vi "LiveData.vi"() -> ()   [LabVIEW 2009]
panel:
  out "error out":errorcluster
  out "Waveform Graph":u16[](graph)
  in  "VISA resource name":refnum<visa-resource-name>="COM21"
  in  "stop":bool
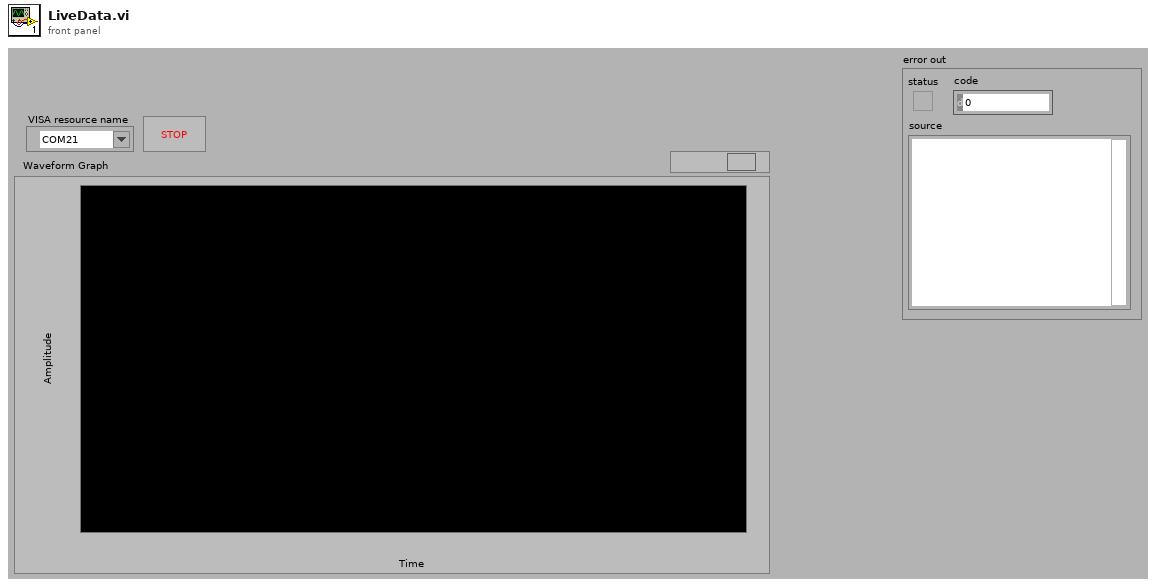
[diagram p1: front panel]
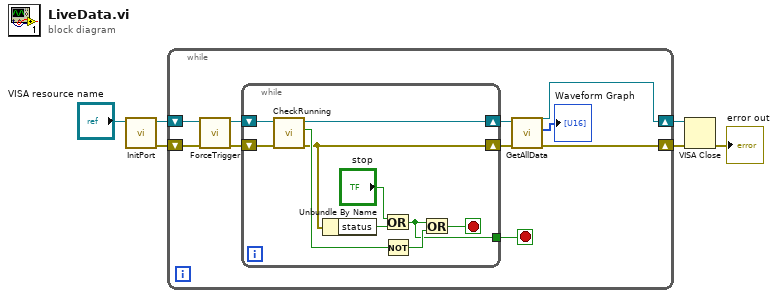
[diagram p0: block diagram]
diagram:
  n1 = call "InitPort.vi"("VISA resource name"="VISA resource name") -> ("error out"=w5:errorcluster, "VISA resource name out"=w4:refnum<visa-resource-name>)  [unwired: 9 in]
  n2 = while {
    shift-right: [w14] -> w3
    shift-left: w4 -> [w16]
    shift-right: [w13] -> w2
    shift-left: w5 -> [w15]
    stop <- w8 stop-if-true
    n3 = call "ForceTrigger.vi"("error in (no error)"=w15, "VISA resource name"=w16) -> ("error out"=w11:errorcluster, "VISA resource name out"=w12:refnum<visa-resource-name>)  [unwired: 8 in]
    n4 = while {
      shift-right: [w26] -> w10
      shift-left: w12 -> [w25]
      shift-right: [w21] -> w9
      shift-left: w11 -> [w24]
      tunnel: [w17] -> w8
      stop <- w19 stop-if-true
      n5 = call "CheckRunning.vi"("error in (no error)"=w24, "VISA resource name"=w25) -> ("error out"=w21:errorcluster, "IsRunning"=w23:bool, "VISA resource name out"=w26:refnum<visa-resource-name>)  [unwired: 7 in]
      n6 = Unbundle By Name(w21) -> ("status"=w20:bool)
      n7 = Or(x="stop", y=w20) -> (x .or. y?=w17:bool)
      n8 = Not(x=w23) -> (.not. x?=w18:bool)
      n9 = Or(x=w17, y=w18) -> (x .or. y?=w19:bool)
    }
    n10 = call "GetAllData.vi"("error In"=w9, "VISA resource In"=w10) -> ("error out"=w13:errorcluster, "Data Out"=→"Waveform Graph":u16[], "VISA resource Out"=w14:refnum<visa-resource-name>)  [unwired: 7 in]
  }
  n11 = VISA Close(VISA resource name=w3, error in (no error)=w2) -> (error out=→"error out":errorcluster)
